vi "PS Control.vi"(11 "Message Enqueuer":refnum<class "Message Enqueuer.lvclass">) -> ()   [LabVIEW 2025]
doc: "Author: Scott Hannahs <sth@magnet.fsu.edu>\n\nThis software is licensed for use under the “MIT License\"\nCopyright (c) 2025 Scott Hannahs, sth@sth@magnet.sthnet.net\n\nPermission is hereby granted, free of charge, to any person obtaining a copy of this software and associated documentation files (the \"Software\"), to deal in the Software without restriction, including without limitation the rights to use, copy, modify, merge, publish, distribute, sublicense, and/or sell copies of the Software, and to permit persons to whom the Software is furnished to do so, subject to the following conditions: The above copyright notice and this permission notice shall be included in all copies or substantial portions of the Software.\n\nTHE SOFTWARE IS PROVIDED \"AS IS\", WITHOUT WARRANTY OF ANY KIND, EXPRESS OR IMPLIED, INCLUDING BUT NOT LIMITED TO THE WARRANTIES OF MERCHANTABILITY, FITNESS FOR A PARTICULAR PURPOSE AND NONINFRINGEMENT. IN NO EVENT SHALL THE AUTHORS OR COPYRIGHT HOLDERS BE LIABLE FOR ANY CLAIM, DAMAGES OR OTHER LIABILITY, WHETHER IN AN ACTION OF CONTRACT, TORT OR OTHERWISE, ARISING FROM, OUT OF OR IN CONNECTION WITH THE SOFTWARE OR THE USE OR OTHER DEALINGS IN THE SOFTWARE."
uses:
  <vilib>/ActorFramework/Message Enqueuer/Message Enqueuer.lvclass
  <vilib>/ActorFramework/Message Enqueuer/Message Enqueuer.lvclass/Message Enqueuer.ctl
  PS Control Actor Messages/Write Staff mode Msg/Write Staff mode Msg.lvclass/Write Staff mode Msg.ctl
  PS Control Actor Messages/Choose configuration mode Msg/Choose configuration mode Msg.lvclass/Choose configuration mode Msg.ctl
  PS Control Actor Messages/Change VISA address Msg/Change VISA address Msg.lvclass/Change VISA address Msg.ctl
  PS Control Actor Messages/Setpoint Msg/Setpoint Msg.lvclass/Setpoint Msg.ctl
  PS Control Actor Messages/RampRate Msg/RampRate Msg.lvclass/RampRate Msg.ctl
  <vilib>/ActorFramework/Message Enqueuer/Enqueue.vi
  PS Control Actor Messages/RampToSetpoint Msg/RampToSetpoint Msg.lvclass
  PS Control Actor Messages/Write Staff mode Msg/Write Staff mode Msg.lvclass
  PS Control Actor Messages/Choose configuration mode Msg/Choose configuration mode Msg.lvclass
  PS Control Actor Messages/Hold Msg/Hold Msg.lvclass
  PS Control Actor Messages/Change VISA address Msg/Change VISA address Msg.lvclass
  PS Control Actor Messages/RampToZero Msg/RampToZero Msg.lvclass
  PS Control Actor Messages/Setpoint Msg/Setpoint Msg.lvclass
  PS Control Actor Messages/RampRate Msg/RampRate Msg.lvclass
  <vilib>/ActorFramework/Stop Msg/Stop Msg.lvclass
  <vilib>/ActorFramework/Message Priority Queue/Priority Enqueue.vi
panel:
  out "Status":string
  in  "Operating mode":u16(ring) items=["SCM1Normal"]
  in  "Staff mode":bool
  out "error out":errorcluster
  in  "VISA address":refnum<visa-resource-name>="GPIB0::22::INSTR"
  in  "stop":bool
  in  "Ramp to Zero":bool
  in  "Hold":bool
  in  "Ramp to Setpoint":bool
  in  "Slew Rate [T/min]":dbl=0.3 format="%_5f"
  in  "Setpoint [T]":dbl format="%.3f"
  out "Magnet\nVoltage":dbl format="%.2f"
  out "Field [T]":dbl format="%.4f"
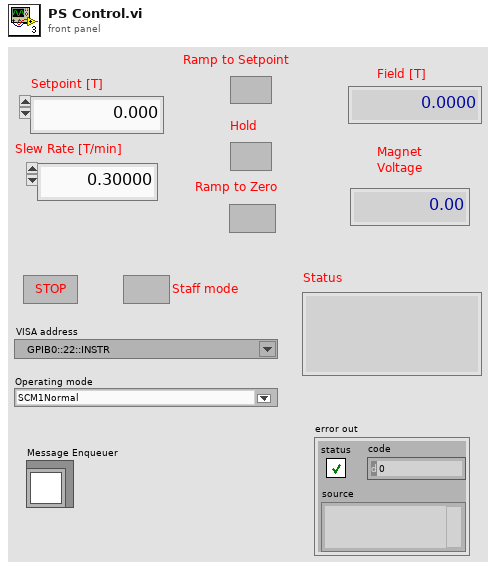
[diagram p1: front panel]
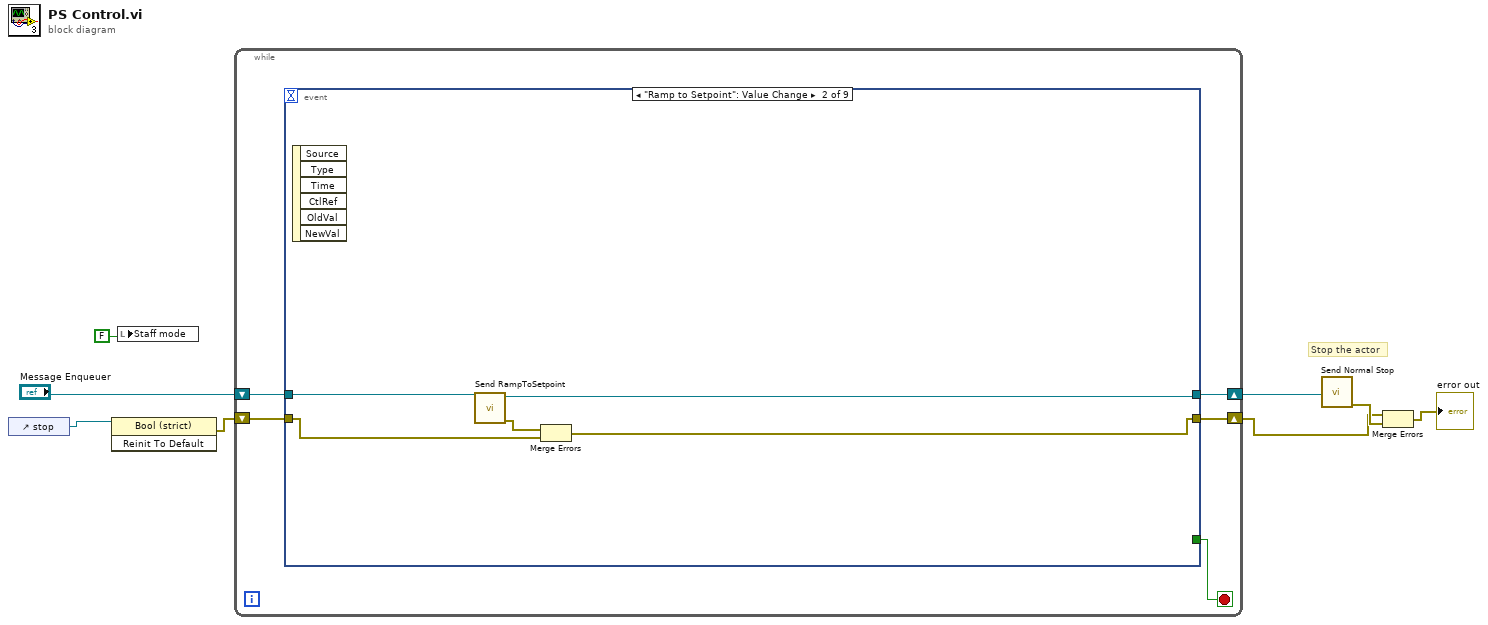
[diagram p0: block diagram]
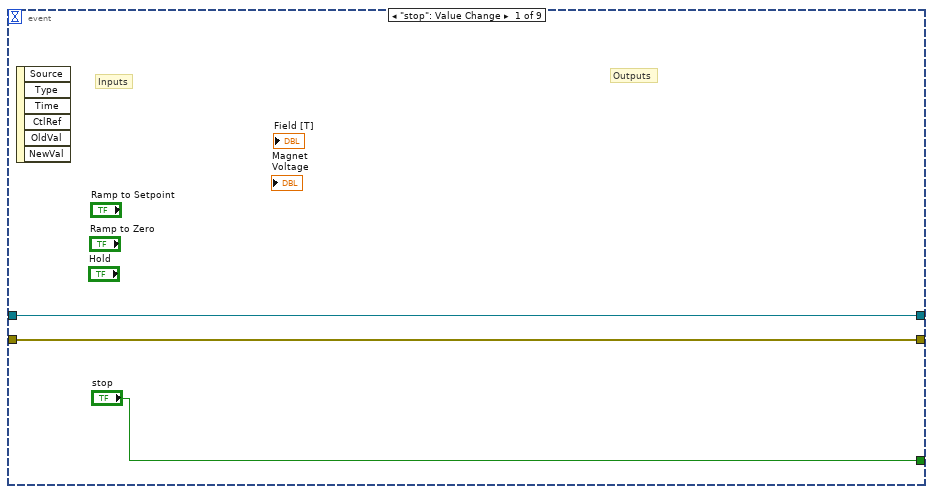
[diagram p2: hidden frame]
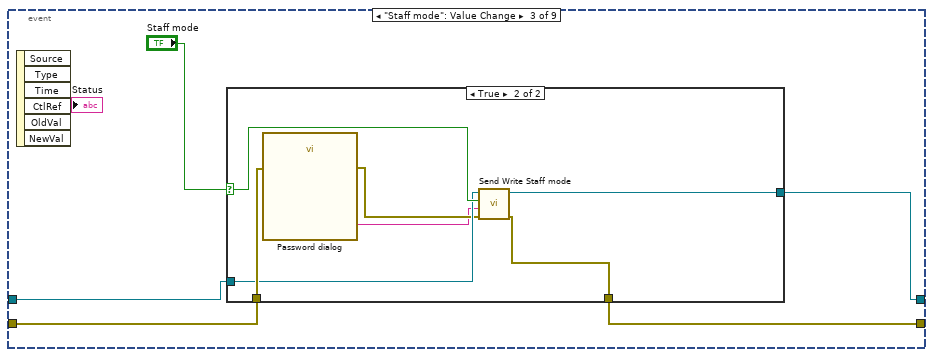
[diagram p3: hidden frame]
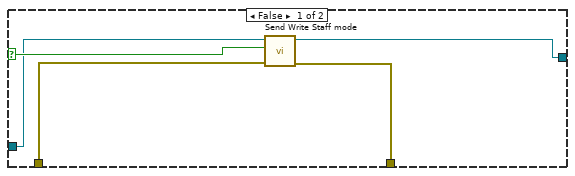
[diagram p4: hidden frame]
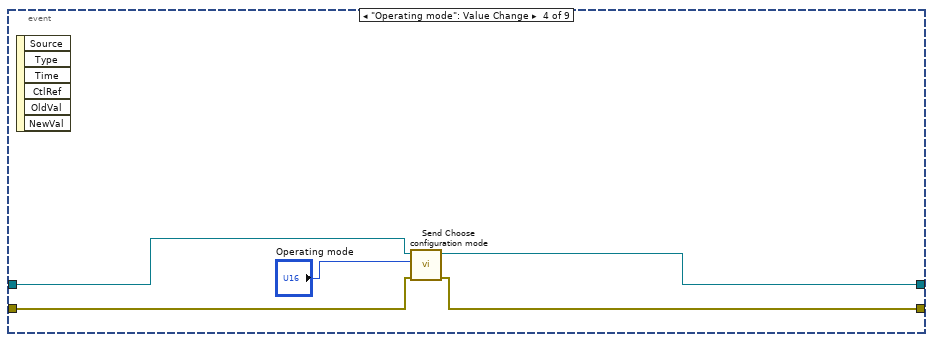
[diagram p5: hidden frame]
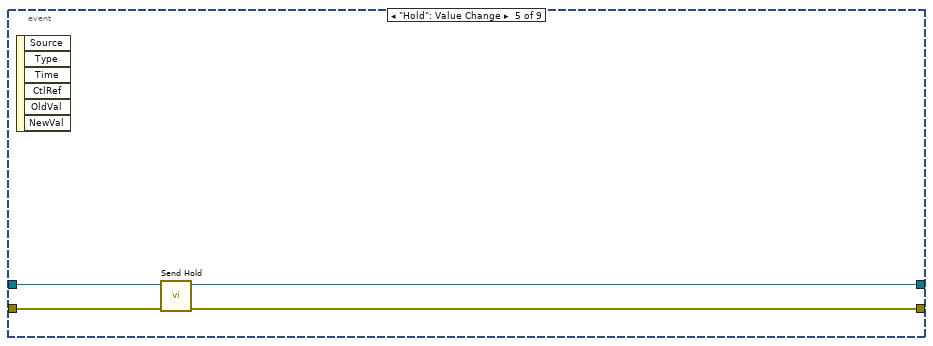
[diagram p6: hidden frame]
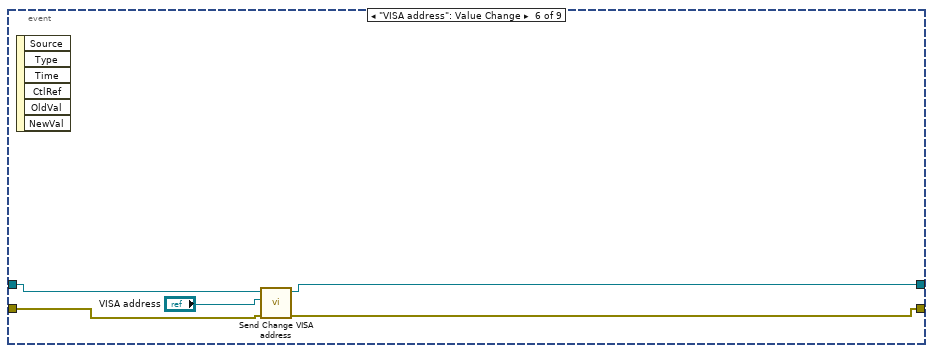
[diagram p7: hidden frame]
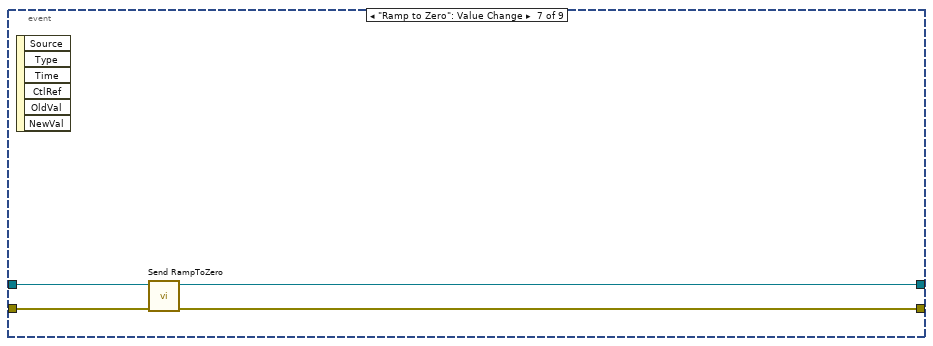
[diagram p8: hidden frame]
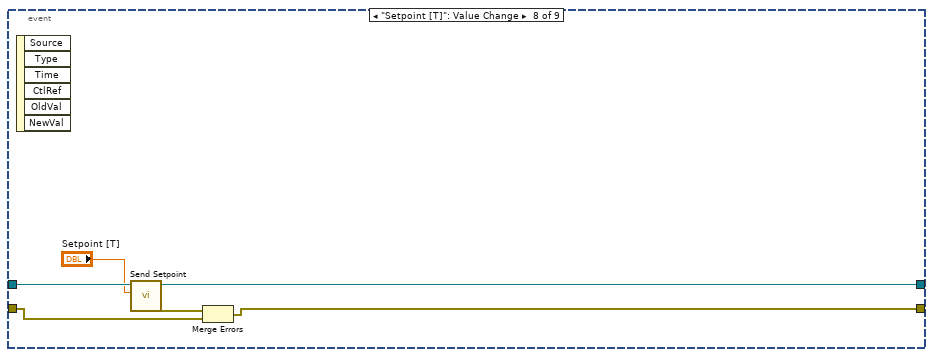
[diagram p9: hidden frame]
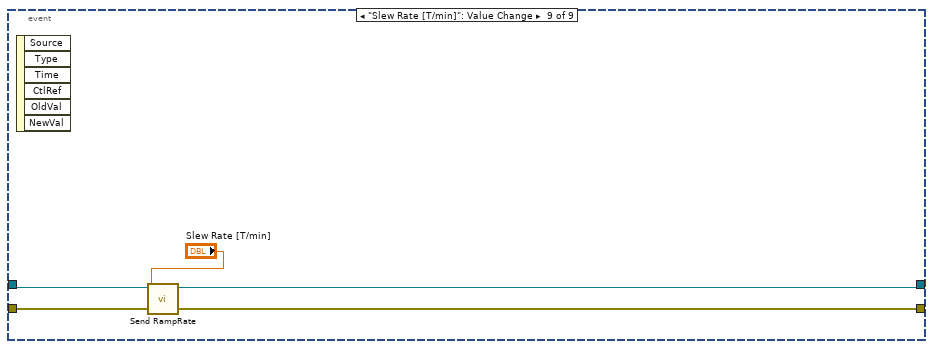
[diagram p10: hidden frame]
diagram:
  # "Stop the actor"
  n1 = control-ref of="stop"() -> (w8:refnum<vi>)
  n2 = invoke class="Bool (strict)" method="Reinit To Default"(reference=w8) -> (error out=w2:errorcluster)  [unwired: 2 in, 2 out]
  n3 = local write "Staff mode"(FALSE ("Staff mode")) -> ()
  n4 = while {
    shift-right: [w10] -> w7
    shift-left: "Message Enqueuer" -> [w12]
    shift-right: [w9] -> w3
    shift-left: w2 -> [w13]
    stop <- w11 stop-if-true
    n5 = event shown="[1] \"Ramp to Setpoint\": Value Change" {
      selector: _ -> [_ _ _ _ _ _ _ _ _]
      dyn-events: _ -> [_ _ _ _ _ _ _ _ _]
      timeout: _ -> [_ _ _ _ _ _ _ _ _]
      tunnel: ["stop" _ _ _ _ _ _ _ _] -> w11
      tunnel: w13 -> [w14 w18 w24 w41 w46 w50 w55 w58 w65]
      tunnel: [w15 w20 w22 w39 w45 w49 w53 w60 w64] -> w10
      tunnel: w12 -> [w15 w21 w23 w42 w47 w51 w56 w62 w66]
      tunnel: [w14 w17 w25 w40 w44 w48 w54 w57 w63] -> w9
      event "stop": Value Change {
        # "Outputs"
        # "Inputs"
        n6 = event-data() -> ()  [unwired: 1 in, 6 out]
      }
      event "Ramp to Setpoint": Value Change {
        n7 = event-data() -> ()  [unwired: 1 in, 6 out]
        n8 = call "Send RampToSetpoint.vi"("Message Enqueuer"=w21) -> ("error out"=w19:errorcluster, "Message Enqueuer out"=w20:refnum<class "Message Enqueuer.lvclass">)  [unwired: 9 in]
        n9 = Merge Errors(w19, w18) -> (w17:errorcluster)
      }
      event "Staff mode": Value Change {
        n10 = event-data() -> ()  [unwired: 1 in, 6 out]
        n11 = case shown="True" "Staff mode" {
          selector: "Staff mode" -> [w30 w37]
          tunnel: [w28 w34] -> w25
          tunnel: w24 -> [w31 w38]
          tunnel: w23 -> [w29 w36]
          tunnel: [w27 w35] -> w22
          frame False {
            n12 = call "Send Write Staff mode.vi"("error in (no error)"=w31, "Staff mode"=w30, "Message Enqueuer"=w29) -> ("error out"=w28:errorcluster, "Message Enqueuer out"=w27:refnum<class "Message Enqueuer.lvclass">)  [unwired: 7 in]
          }
          frame True {
            n13 = call "Password dialog.vi"("error in (no error)"=w38) -> ("Password"=w32:string, "error out"=w33:errorcluster)  [unwired: 16 in, 1 out]
            n14 = call "Send Write Staff mode.vi"("error in (no error)"=w33, "Password"=w32, "Staff mode"=w37, "Message Enqueuer"=w36) -> ("error out"=w34:errorcluster, "Message Enqueuer out"=w35:refnum<class "Message Enqueuer.lvclass">)  [unwired: 6 in]
          }
        }
      }
      event "Operating mode": Value Change {
        n15 = event-data() -> ()  [unwired: 1 in, 6 out]
        n16 = call "Send Choose configuration mode.vi"("error in (no error)"=w41, "Choose configuration mode"="Operating mode", "Message Enqueuer"=w42) -> ("error out"=w40:errorcluster, "Message Enqueuer out"=w39:refnum<class "Message Enqueuer.lvclass">)  [unwired: 7 in]
      }
      event "Hold": Value Change {
        n17 = event-data() -> ()  [unwired: 1 in, 6 out]
        n18 = call "Send Hold.vi"("error in (no error)"=w46, "Message Enqueuer"=w47) -> ("error out"=w44:errorcluster, "Message Enqueuer out"=w45:refnum<class "Message Enqueuer.lvclass">)  [unwired: 8 in]
      }
      event "VISA address": Value Change {
        n19 = event-data() -> ()  [unwired: 1 in, 6 out]
        n20 = call "Send Change VISA address.vi"("error in (no error)"=w50, "VISA address"="VISA address", "Message Enqueuer"=w51) -> ("error out"=w48:errorcluster, "Message Enqueuer out"=w49:refnum<class "Message Enqueuer.lvclass">)  [unwired: 7 in]
      }
      event "Ramp to Zero": Value Change {
        n21 = event-data() -> ()  [unwired: 1 in, 6 out]
        n22 = call "Send RampToZero.vi"("error in (no error)"=w55, "Message Enqueuer"=w56) -> ("error out"=w54:errorcluster, "Message Enqueuer out"=w53:refnum<class "Message Enqueuer.lvclass">)  [unwired: 8 in]
      }
      event "Setpoint [T]": Value Change {
        n23 = event-data() -> ()  [unwired: 1 in, 6 out]
        n24 = call "Send Setpoint.vi"("Setpoint [T]"="Setpoint [T]", "Message Enqueuer"=w62) -> ("error out"=w59:errorcluster, "Message Enqueuer out"=w60:refnum<class "Message Enqueuer.lvclass">)  [unwired: 8 in]
        n25 = Merge Errors(w59, w58) -> (w57:errorcluster)
      }
      event "Slew Rate [T/min]": Value Change {
        n26 = event-data() -> ()  [unwired: 1 in, 6 out]
        n27 = call "Send RampRate.vi"("error in (no error)"=w65, "Ramp rate (T/min)"="Slew Rate [T/min]", "Message Enqueuer"=w66) -> ("error out"=w63:errorcluster, "Message Enqueuer out"=w64:refnum<class "Message Enqueuer.lvclass">)  [unwired: 7 in]
      }
    }
  }
  n28 = call <vilib>:"Send Normal Stop.vi"("Message Enqueuer"=w7) -> ("error out"=w4:errorcluster)  [unwired: 10 in]
  n29 = Merge Errors(w3, w4) -> (→"error out":errorcluster)
